vi "NI Test Server Only Bound Variable Read-Write.vi"() -> ()   [LabVIEW 2011]
doc: "This Arbitrary Waveform Generator front panel is aimed primarily at the use of two reflectometer instruments at the ISIS Pulsed Neutron Facility at the Rutherford Appleton Laboratory. As such some variable items have been defaulted, and the code follows the standards of the Instrument Controls programming team."
uses:
  Labview Modules/Common/Utilities/Logo.llb/Logo.ctl
  Labview Modules/Common/Utilities/VI Control.llb/Control - Display State.ctl
  Labview Modules/Drivers/Tektronix AFG 3021B/AFG3021B - Controls.llb/AFG3021B - Trigger Button.ctl
  Labview Modules/Common/Utilities/Equal.llb/Equal - Error.vi
panel:
  out "Set Point Ind":dbl
  in  "Set Point":dbl
  in  "Exit":bool
  in  "Set":bool
  out "Message":string
  out "Activity":bool
  out "Error":errorcluster
  in  "Logo":T1
  # "Version 0.0.1"
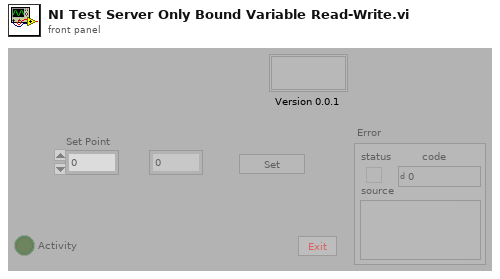
[diagram p1: front panel]
types:
  T1 = typedef "Logo.ctl" = u16
  T2 = typedef "Control - Display State.ctl" = enum16{"Enabled", "Disabled", "Disabled and Grayed"}
  T3 = typedef "AFG3021B - Trigger Button.ctl" = bool
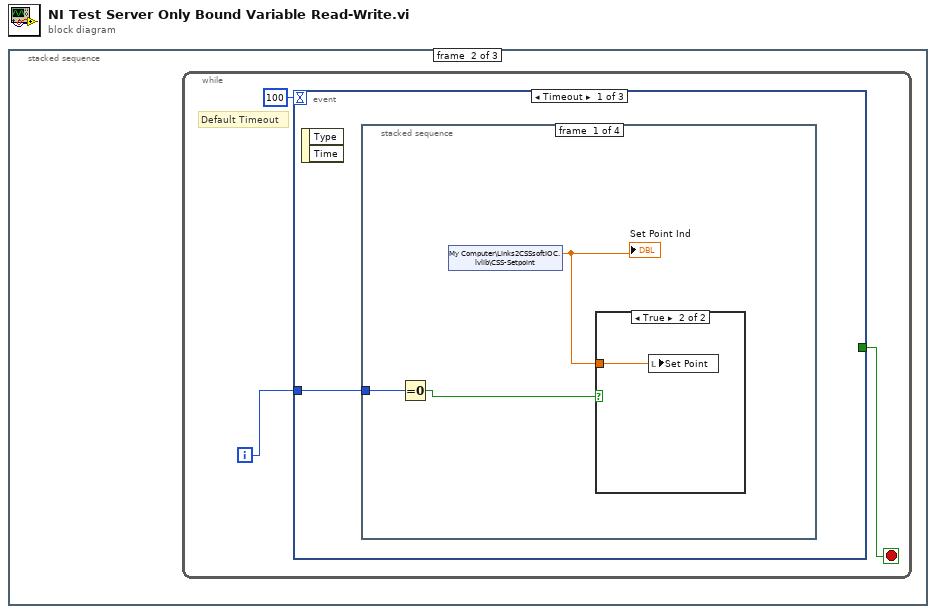
[diagram p0: block diagram]
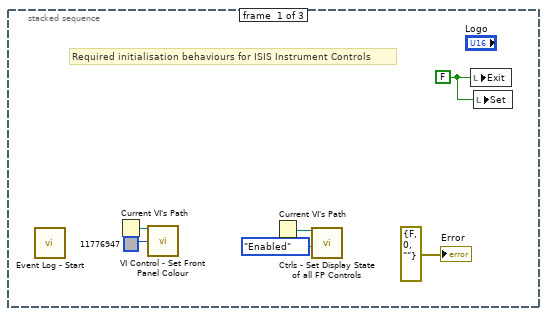
[diagram p2: hidden frame]
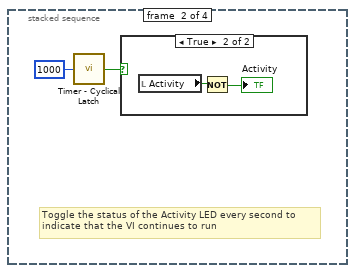
[diagram p4: hidden frame]
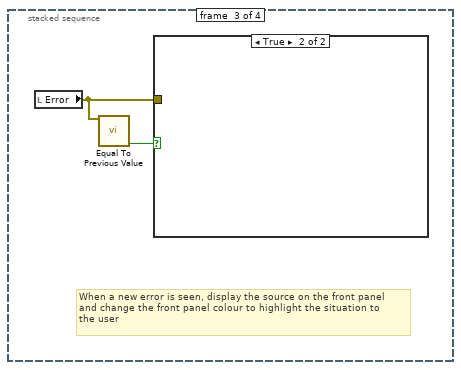
[diagram p6: hidden frame]
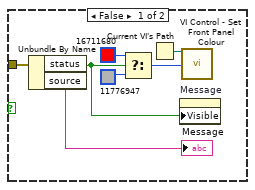
[diagram p7: hidden frame]
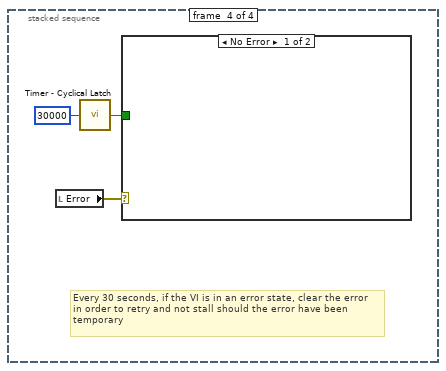
[diagram p8: hidden frame]
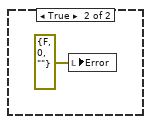
[diagram p10: hidden frame]
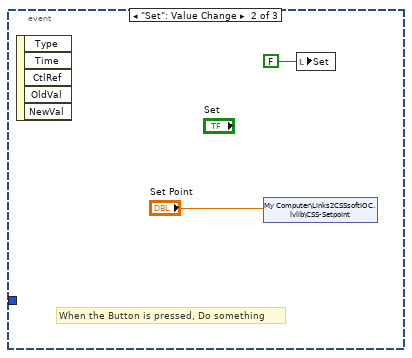
[diagram p11: hidden frame]
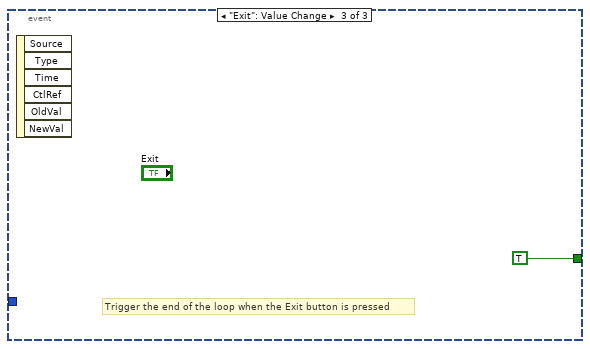
[diagram p12: hidden frame]
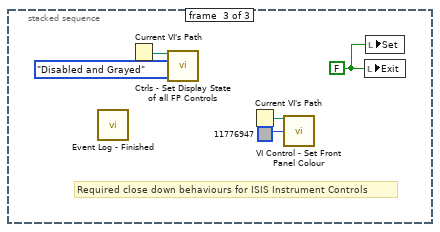
[diagram p13: hidden frame]
diagram:
  n1 = stacked-sequence {
    frame #0 {
      w1 = FALSE
      # "Required initialisation behaviours for ISIS Instrument Controls"
      n2 = call "Event Log - Start.vi"() -> ()  [unwired: 1 in]
      n3 = Current VI's Path() -> (path=w2:path)
      n4 = call "VI Control - Set Front Panel Colour.vi"("VI Path"=w2, "Front Panel Colour"=u32 11776947) -> ()  [unwired: 13 in, 1 out]
      n5 = Current VI's Path() -> (path=w6:path)
      n6 = call "Ctrls - Set Display State of all FP Controls.vi"("VI Path"=w6, "Display State"=Control_-_Display_State."Enabled") -> ()  [unwired: 18 in]
      n7 = local write "Exit"(w1) -> ()
      n8 = local write "Set"(w1) -> ()
      "Error" <- errorcluster {"status"=FALSE, "code"=0, "source"=""} ("Error")
    }
    frame #1 {
      n9 = while {
        i -> [w7]
        stop <- w8 stop-if-true
        # "Default Timeout"
        n10 = event shown="[0] Timeout" {
          selector: _ -> [_ _ _]
          dyn-events: _ -> [_ _ _]
          timeout: 100 -> [_ _ _]
          tunnel: [_ _ TRUE] -> w8
          tunnel: w7 -> [w10 _ _]
          event Timeout {
            n11 = event-data() -> ()  [unwired: 1 in, 2 out]
            n12 = stacked-sequence {
              tunnel: w10 -> [w13 _ _ _]
              frame #0 {
                n13 = Equal To 0?(x=w13) -> (x = 0?=w12:bool)
                n14 = shared-variable "My Computer\\Links2CSSsoftIOC.lvlib\\CSS-Setpoint"() -> (w11:dbl)  [unwired: 1 in, 1 out]
                "Set Point Ind" <- w11
                n15 = case shown="True" w12 {
                  tunnel: w11 -> [_ w14]
                  frame False {
                  }
                  frame True {
                    n16 = local write "Set Point"(w14) -> ()
                  }
                }
              }
              frame #1 {
                # "Toggle the status of the Activity LED every second to\nindicate that the VI continues to run"
                n17 = call "Timer - Cyclical Latch.vi"("Timer (msec)"=u32 1000) -> ("Timer Trigger"=w15:bool)  [unwired: 14 in]
                n18 = case shown="True" w15 {
                  frame False {
                  }
                  frame True {
                    n19 = local read "Activity"() -> (w17:bool)
                    n20 = Not(x=w17) -> (.not. x?=→"Activity":bool)
                  }
                }
              }
              frame #2 {
                # "When a new error is seen, display the source on the front panel\nand change the front panel colour to highlight the situation to\nthe user"
                n21 = local read "Error"() -> (w20:errorcluster)
                n22 = call-poly "Equal To Previous Value.vi"("Value In"=w20) -> ("Equal to previous value"=w19:bool)  [unwired: 13 in, 1 out]
                n23 = case shown="True" w19 {
                  tunnel: w20 -> [w23 _]
                  frame False {
                    n24 = Unbundle By Name(w23) -> ("status"=w22:bool, "source"=→"Message":string)
                    n25 = Select(t=u32 16711680, s=w22, f=u32 11776947) -> (s? t:f=w24:u32)
                    n26 = Current VI's Path() -> (path=w27:path)
                    n27 = property on="Message" class="Str"("Visible"=w22) -> ()  [unwired: 2 in, 2 out]
                    n28 = call "VI Control - Set Front Panel Colour.vi"("VI Path"=w27, "Front Panel Colour"=w24) -> ()  [unwired: 13 in, 1 out]
                  }
                  frame True {
                  }
                }
              }
              frame #3 {
                # "Every 30 seconds, if the VI is in an error state, clear the error\nin order to retry and not stall should the error have been \ntemporary"
                n29 = local read "Error"() -> (w29:errorcluster)
                n30 = call "Timer - Cyclical Latch.vi"("Timer (msec)"=u32 30000) -> ("Timer Trigger"=w28:bool)  [unwired: 14 in]
                n31 = case shown="No Error" w29 {
                  tunnel: w28 -> [_ w31]
                  frame No Error {
                  }
                  frame Error {
                    n32 = case shown="False" w31 {
                      frame False {
                      }
                      frame True {
                        n33 = local write "Error"(errorcluster {"status"=FALSE, "code"=0, "source"=""} ("Error")) -> ()
                      }
                    }
                  }
                }
              }
            }
          }
          event "Set": Value Change {
            # "When the Button is pressed, Do something"
            n34 = event-data() -> ()  [unwired: 1 in, 5 out]
            n35 = shared-variable "My Computer\\Links2CSSsoftIOC.lvlib\\CSS-Setpoint"("Set Point") -> ()  [unwired: 1 in, 1 out]
            n36 = local write "Set"(T3 FALSE ("Trigger")) -> ()
          }
          event "Exit": Value Change {
            # "Trigger the end of the loop when the Exit button is pressed"
            n37 = event-data() -> ()  [unwired: 1 in, 6 out]
          }
        }
      }
    }
    frame #2 {
      w36 = FALSE
      # "Required close down behaviours for ISIS Instrument Controls"
      n38 = call "Event Log - Finished.vi"() -> ()  [unwired: 1 in]
      n39 = Current VI's Path() -> (path=w39:path)
      n40 = call "Ctrls - Set Display State of all FP Controls.vi"("VI Path"=w39, "Display State"=Control_-_Display_State."Disabled and Grayed") -> ()  [unwired: 18 in]
      n41 = Current VI's Path() -> (path=w38:path)
      n42 = call "VI Control - Set Front Panel Colour.vi"("VI Path"=w38, "Front Panel Colour"=u32 11776947) -> ()  [unwired: 13 in, 1 out]
      n43 = local write "Exit"(w36) -> ()
      n44 = local write "Set"(w36) -> ()
    }
  }
